vi "Get Chassis Info.vi"(8 "error in":errorcluster, 9 "System Hardware":refnum<k20>, 11 "SysAPI Session":refnum<k21>) -> (0 "error out":errorcluster, 1 "System Hardware":refnum<k20>, 2 "IP Address":string, 3 "SysAPI Session":refnum<k21>, 5 "Device Connected?":bool, 7 "ChassisType":T1=enum."C Series 1-Slot")   [LabVIEW 2012]
uses:
  Common/Controls/Chassis Type.ctl
  <resource>/objmgr/nisysapi.rc
  Cfg Grandmaster.lvclass
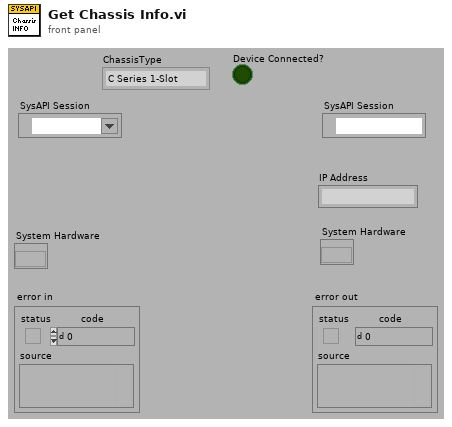
[diagram p1: front panel]
types:
  T1 = typedef "Chassis Type.ctl" = enum16{"Not Supported", "C Series 1-Slot", "C Series 4-Slot", "C Series 8-Slot", "PXI 8-Slot", "PXIe 18-Slot"}
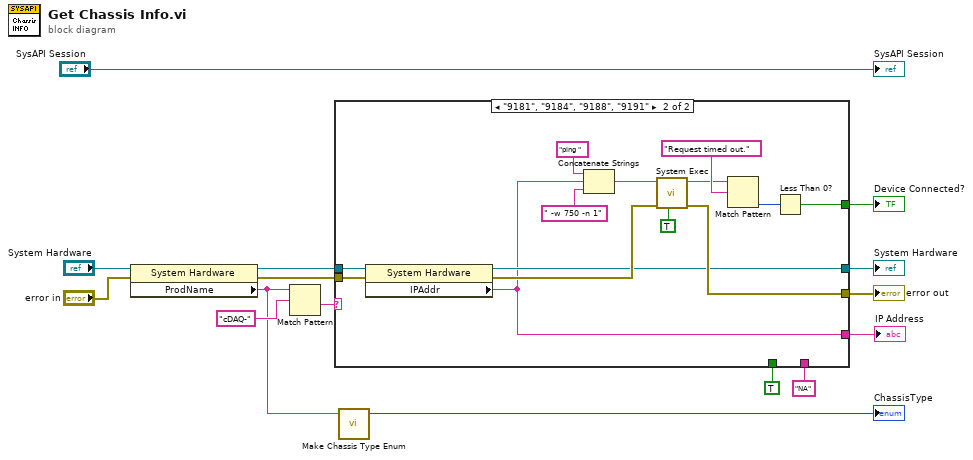
[diagram p0: block diagram]
diagram:
  n1 = property class="System Hardware"(reference="System Hardware", error in="error in") -> (reference out=w4:refnum<k20>, error out=w11:errorcluster, "ProdName"=w6:string)
  n2 = Match Pattern(string=w6, regular expression="cDAQ-") -> (after substring=w12:string)  [unwired: 1 in, 3 out]
  n3 = case shown="\"9181\", \"9184\", \"9188\", \"9191\"" w12 {
    tunnel: [w18 w33] -> w15
    tunnel: [w19 w32] -> w14
    tunnel: w11 -> [w19 w24]
    tunnel: TRUE -> [w18 _]
    tunnel: w4 -> [w17 w23]
    tunnel: [w17 w21] -> w3
    tunnel: [w16 w20] -> w2
    tunnel: "NA" ("IPAddr") -> [w16 _]
    frame Default {
    }
    frame "9181", "9184", "9188", "9191" {
      n4 = property class="System Hardware"(reference=w23, error in=w24) -> (reference out=w21:refnum<k20>, error out=w22:errorcluster, "IPAddr"=w20:string)
      n5 = Concatenate Strings("ping " ("command line"), w20, " -w 750 -n 1" ("command line")) -> (w25:string)
      n6 = call <vilib>:"System Exec.vi"("run minimized? (F)"=TRUE, "error in (no error)"=w22, "command line"=w25) -> ("error out"=w32:errorcluster, "standard output"=w29:string)  [unwired: 5 in, 2 out]
      n7 = Match Pattern(string=w29, regular expression="Request timed out.") -> (offset past match=w28:i32)  [unwired: 1 in, 3 out]
      n8 = Less Than 0?(x=w28) -> (x < 0?=w33:bool)
    }
  }
  "Device Connected?" <- w15
  "error out" <- w14
  "System Hardware" <- w3
  "IP Address" <- w2
  n9 = call "Make Chassis Type Enum.vi"("ProductType"=w6) -> ("ChassisType"=→"ChassisType":T1)  [unwired: 4 in]
  "SysAPI Session" <- "SysAPI Session"
